vi "Periodic Tasks.vi"(8 "error in":errorcluster) -> ()   [LabVIEW 2020]
doc: "This VI runs in parallel to other tasks. It can contain as many user-defined periodic loops as you need. These can carry out PID or other sorts of timed response."
uses:
  <vilib>/Rock Robotics/WPI/Utilities/WPI_GetSetVariantRefNum.vi
  Robot sans CAN/MyGlobal.vi
  <vilib>/Rock Robotics/Network Tables/NT Write Numeric Array.vi
panel:
  out "force moteurs lance balle":dbl
  out "force feed balle":dbl
  out "ramasse balle":dbl
  out "Deploiement ramasse balle":dbl
  out "winch":dbl
  out "winch 2":dbl
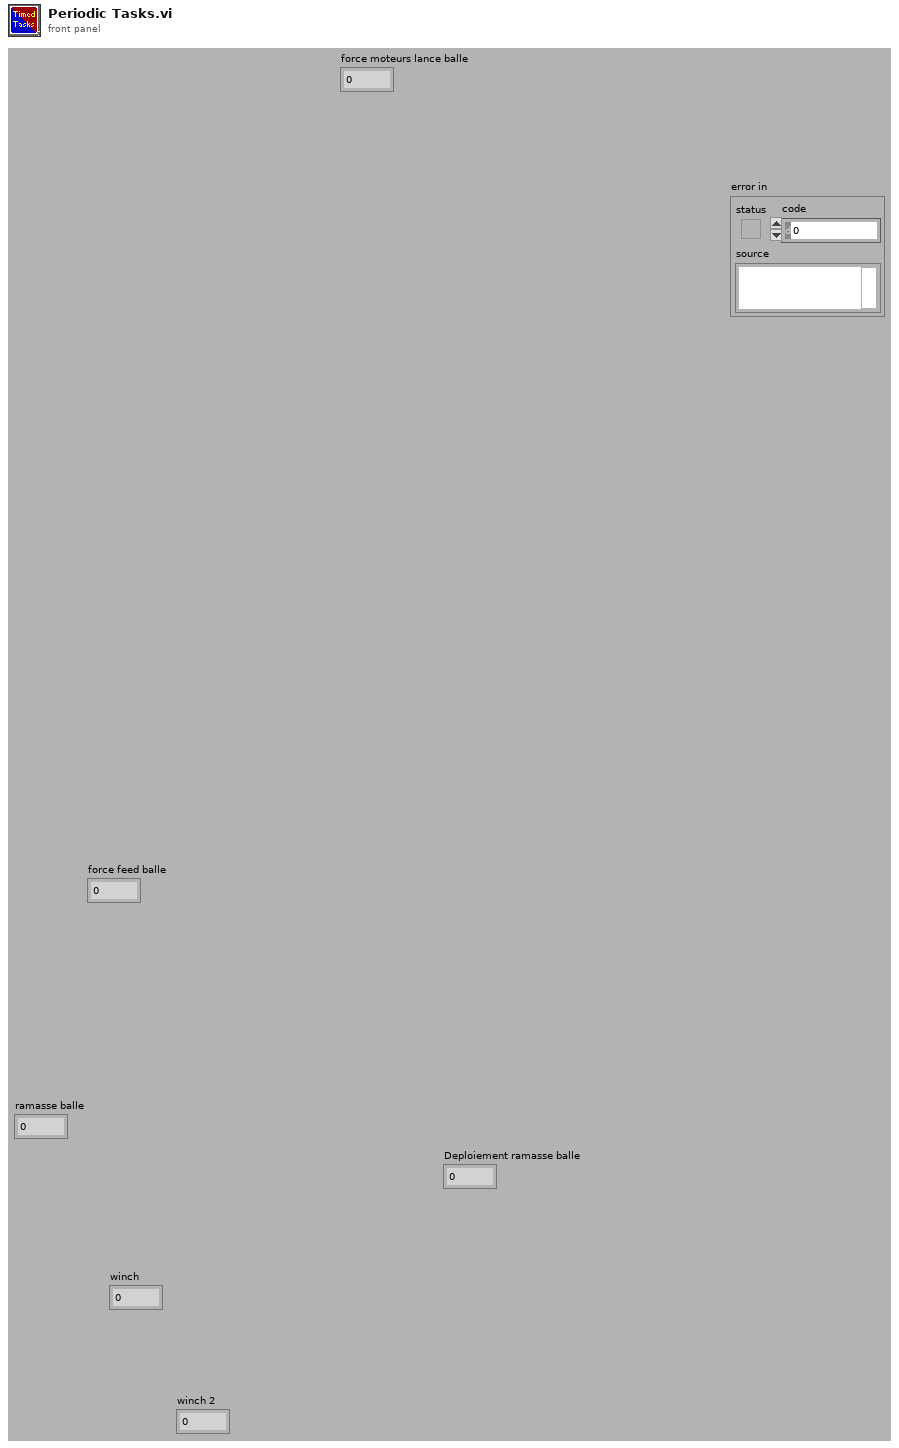
[diagram p1: front panel]
types:
  T1 = typedef "WPI_JoystickDevRef.ctl" = cluster{"Device":T2}
  T2 = typedef "WPI_JoystickDeviceEnum.ctl" = enum16{"USB 0", "USB 1", "USB 2", "USB 3", "USB 4", "USB 5"}
  T3 = typedef "WPI_RobotDriveDevRef.ctl" = cluster{"DevStatus":errorcluster, "Motors[]":T4[], "Square Inputs":bool, "Max Output":dbl}
  T4 = typedef "WPI_MotorControlDeviceRef.ctl" = cluster{"DeviceStatus":errorcluster, "Type":T5, "PWM":cluster{"PWM Channel":T6, "DeadBand":T7}, "CAN":cluster{"Device Number":u8, "SetOutput VI Ref":variant, "GetOutput VI Ref":variant, "Enable VI Ref":variant, "Disable VI Ref":variant, "Data":variant}, "Invert":bool, "DIO PWM":cluster{"PWM \"Enable\" Channel":T6, "DIOChannel":T8, "PWM Rate":dbl}}
  T5 = typedef "WPI_MotorControlType.ctl" = enum16{"PWM", "CAN", "DIO PWM"}
  T6 = typedef "FPGA_DIOPWMChannel.ctl" = enum8{"PWM 0", "PWM 1", "PWM 2", "PWM 3", "PWM 4", "PWM 5", "PWM 6", "PWM 7", "PWM 8", "PWM 9", "PWM MXP 0", "PWM MXP 1", "PWM MXP 2", "PWM MXP 3", "PWM MXP 4", "PWM MXP 5", "PWM MXP 6", "PWM MXP 7", "PWM MXP 8", "PWM MXP 9", "Invalid"}
  T7 = typedef "WPI_PWMDeadband.ctl" = cluster{"Name":string, "maxPositivePwm":i32, "minPositivePwm":i32, "centerPwm":i32, "maxNegativePwm":i32, "minNegativePwm":i32, "angularRange":u16}
  T8 = typedef "FPGA_DIOChannel.ctl" = enum8{"DIO 0", "DIO 1", "DIO 2", "DIO 3", "DIO 4", "DIO 5", "DIO 6", "DIO 7", "DIO 8", "DIO 9", "DIO MXP 0", "DIO MXP 1", "DIO MXP 2", "DIO MXP 3", "DIO MXP 4", "DIO MXP 5", "DIO MXP 6", "DIO MXP 7", "DIO MXP 8", "DIO MXP 9", "DIO MXP 10", "DIO MXP 11", "DIO MXP 12", "DIO MXP 13", "DIO MXP 14", "DIO MXP 15", "SPI Port CS1", "SPI Port CS2", "SPI Port CS3", "SPI Port MISO", "SPI Port MOSI", "Invalid"}
  T9 = cluster{"JoystickDevRef":T1, "RobotDriveDevRef":T3}
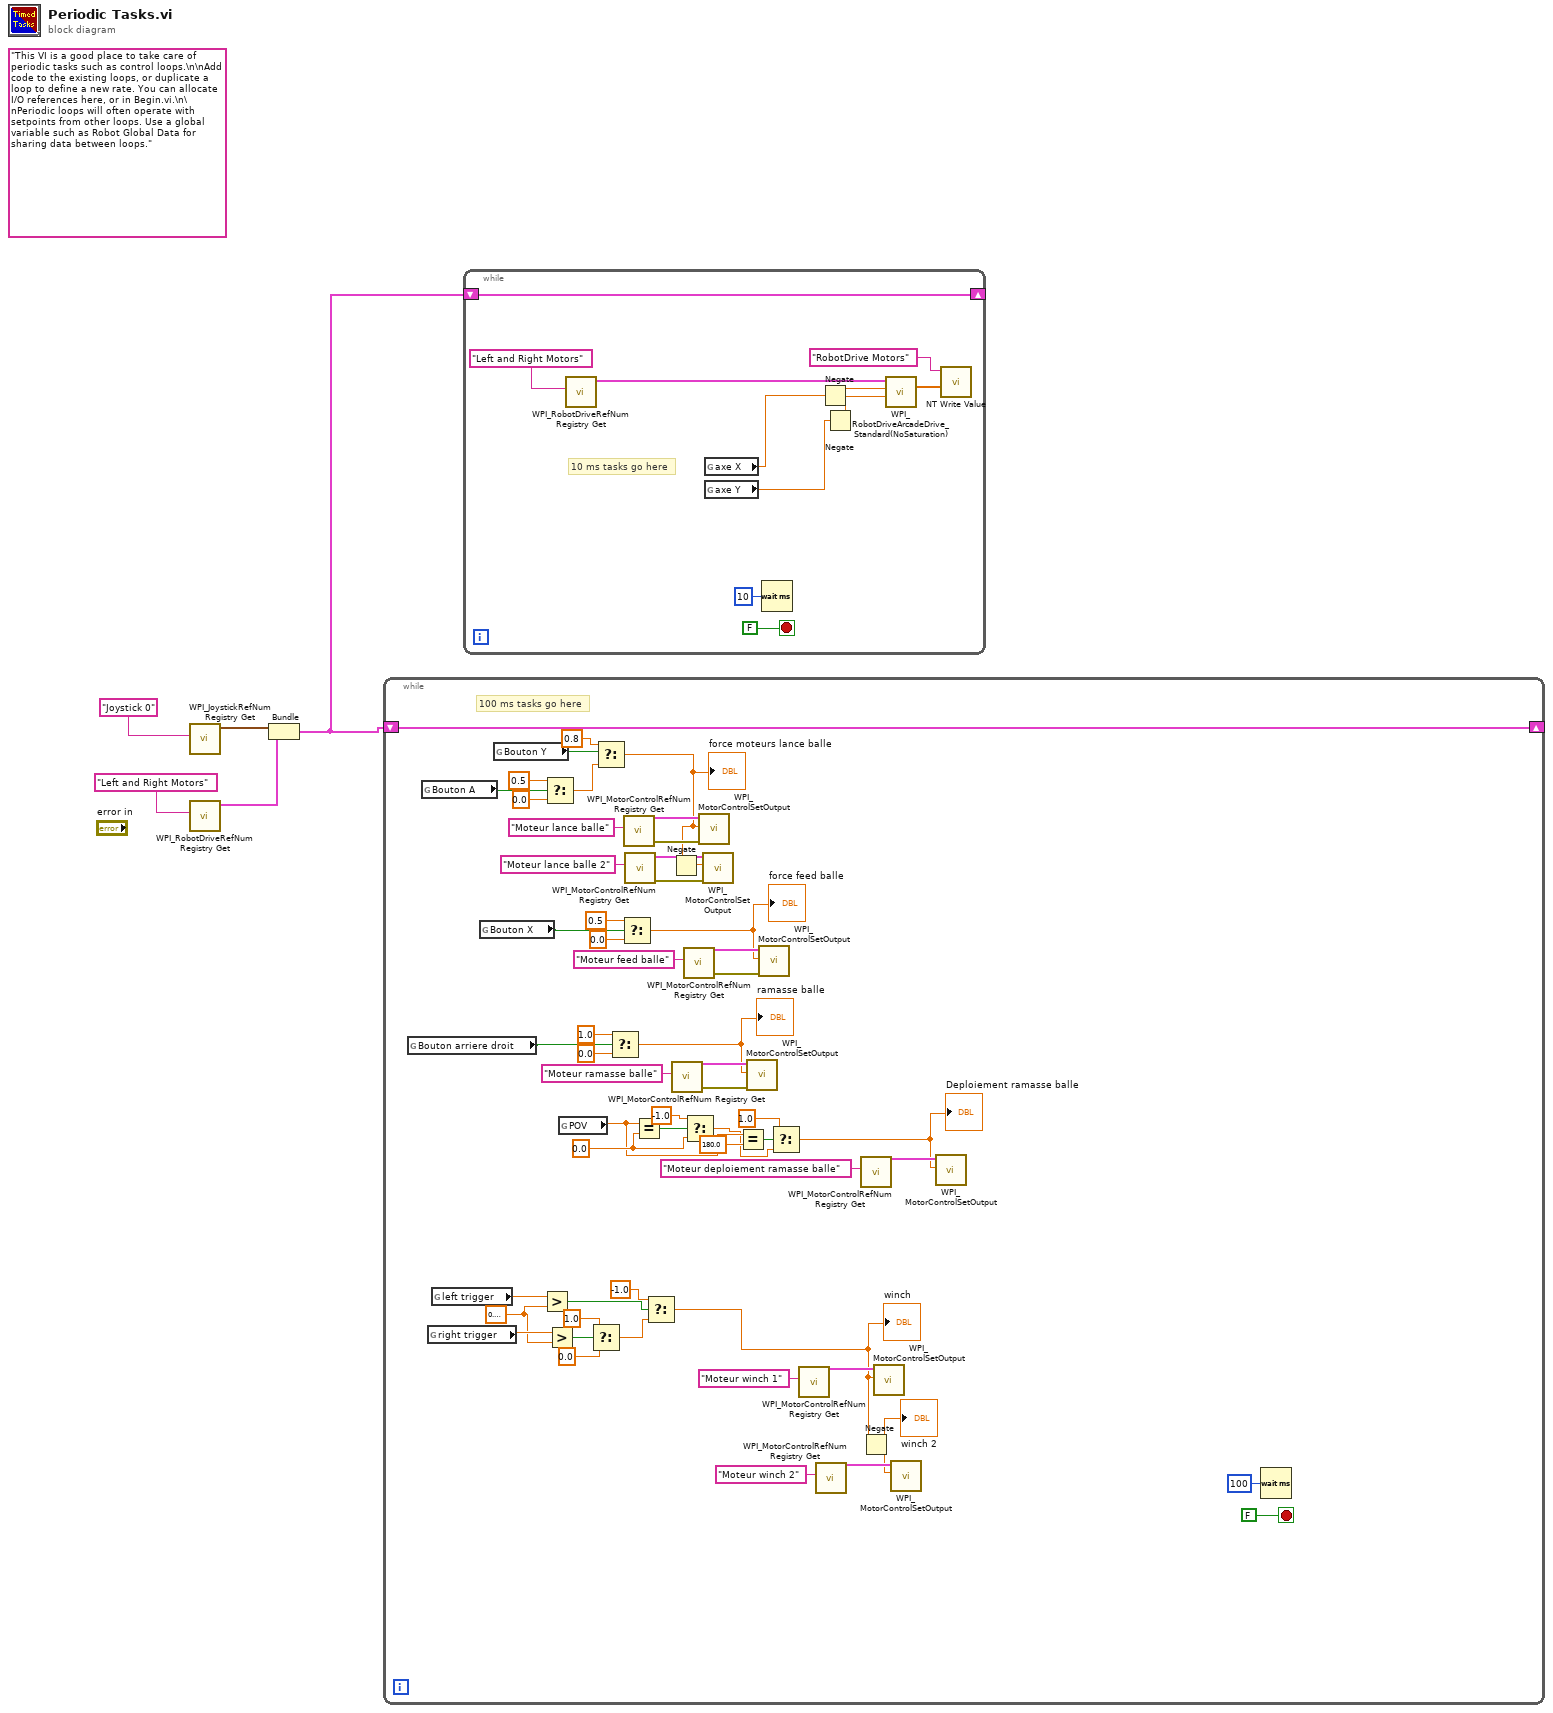
[diagram p0: block diagram]
diagram:
  (unwired) "This VI is a good place to take care of periodic tasks such as control loops.\n\nAdd code to the existing loops, or duplicate a loop to define a new rate. You can allocate I/O references here, or in Begin.vi.\n\nPeriodic loops will often operate with setpoints from other loops. Use a global variable such as Robot Global Data for sharing data between loops."
  n1 = call <vilib>:"WPI_JoystickRefNum Registry Get.vi"("refnum name"="Joystick 0") -> ("JoystickDevRef"=w3:T1)  [unwired: 1 in, 9 out]
  n2 = call <vilib>:"WPI_RobotDriveRefNum Registry Get.vi"("refnum name"="Left and Right Motors") -> ("RobotDriveDevRef"=w2:T3)  [unwired: 1 in, 9 out]
  n3 = Bundle("JoystickDevRef"=w3, "RobotDriveDevRef"=w2) -> (w1:T9)  [unwired: 1 out]
  n4 = while {
    shift-right: [w60] -> _
    shift-left: w1 -> [w60]
    stop <- FALSE stop-if-true
    w18 = sgl 0.2 ("y")
    w29 = 0.0
    # "100 ms tasks go here"
    n5 = global read "MyGlobal.vi" "Bouton arriere droit"() -> (w32:bool)
    n6 = global read "MyGlobal.vi" "Bouton A"() -> (w59:bool)
    n7 = global read "MyGlobal.vi" "right trigger"() -> (w19:sgl)
    n8 = global read "MyGlobal.vi" "left trigger"() -> (w20:sgl)
    n9 = global read "MyGlobal.vi" "Bouton X"() -> (w43:bool)
    n10 = global read "MyGlobal.vi" "Bouton Y"() -> (w55:bool)
    n11 = Greater?(x=w20, y=w18) -> (0:w15:bool)
    n12 = Select(t=0.5, s=w59, f=0.0) -> (s? t:f=w54:dbl)
    n13 = Greater?(x=w19, y=w18) -> (0:w17:bool)
    n14 = global read "MyGlobal.vi" "POV"() -> (w27:sgl)
    n15 = Select(t=1.0, s=w17, f=0.0) -> (s? t:f=w16:dbl)
    n16 = Select(t=0.8, s=w55, f=w54) -> (s? t:f=w47:dbl)
    "force moteurs lance balle" <- w47
    n17 = Select(t=1.0, s=w32, f=0.0) -> (s? t:f=w33:dbl)
    "ramasse balle" <- w33
    n18 = Select(t=0.5, s=w43, f=0.0) -> (s? t:f=w39:dbl)
    "force feed balle" <- w39
    n19 = call <vilib>:"WPI_MotorControlRefNum Registry Get.vi"("refnum name"="Moteur lance balle") -> ("error out"=w50:errorcluster, "MotorControlDevRef"=w51:T4)  [unwired: 9 in]
    n20 = call <vilib>:"WPI_MotorControlRefNum Registry Get.vi"("refnum name"="Moteur lance balle 2") -> ("error out"=w48:errorcluster, "MotorControlDevRef"=w49:T4)  [unwired: 9 in]
    n21 = Equal?(x=w27, y=w29) -> (x = y?=w31:bool)
    n22 = Select(t=-1.0, s=w15, f=w16) -> (s? t:f=w7:dbl)
    "winch" <- w7
    n23 = Negate(x=w47) -> (-x=w46:dbl)
    n24 = call <vilib>:"WPI_MotorControlRefNum Registry Get.vi"("refnum name"="Moteur ramasse balle") -> ("error out"=w34:errorcluster, "MotorControlDevRef"=w35:T4)  [unwired: 9 in]
    n25 = call <vilib>:"WPI_MotorControlRefNum Registry Get.vi"("refnum name"="Moteur feed balle") -> ("error out"=w40:errorcluster, "MotorControlDevRef"=w41:T4)  [unwired: 9 in]
    n26 = Select(t=-1.0, s=w31, f=w29) -> (s? t:f=w24:dbl)
    n27 = call <vilib>:"WPI_MotorControlSetOutput.vi"("error in (no error)"=w50, "Output"=w47, "MotorControlDevRef"=w51) -> ()  [unwired: 6 in, 3 out]
    n28 = call <vilib>:"WPI_MotorControlSetOutput.vi"("error in (no error)"=w48, "Output"=w46, "MotorControlDevRef"=w49) -> ()  [unwired: 6 in, 3 out]
    n29 = Equal?(x=w27, y=sgl 180.0) -> (x = y?=w28:bool)
    n30 = call <vilib>:"WPI_MotorControlSetOutput.vi"("error in (no error)"=w34, "Output"=w33, "MotorControlDevRef"=w35) -> ()  [unwired: 6 in, 3 out]
    n31 = call <vilib>:"WPI_MotorControlSetOutput.vi"("error in (no error)"=w40, "Output"=w39, "MotorControlDevRef"=w41) -> ()  [unwired: 6 in, 3 out]
    n32 = Select(t=1.0, s=w28, f=w24) -> (s? t:f=w21:dbl)
    "Deploiement ramasse balle" <- w21
    n33 = call <vilib>:"WPI_MotorControlRefNum Registry Get.vi"("refnum name"="Moteur winch 1") -> ("MotorControlDevRef"=w10:T4)  [unwired: 9 in, 1 out]
    n34 = call <vilib>:"WPI_MotorControlRefNum Registry Get.vi"("refnum name"="Moteur winch 2") -> ("MotorControlDevRef"=w8:T4)  [unwired: 9 in, 1 out]
    n35 = call <vilib>:"WPI_MotorControlRefNum Registry Get.vi"("refnum name"="Moteur deploiement ramasse balle") -> ("MotorControlDevRef"=w22:T4)  [unwired: 9 in, 1 out]
    n36 = Negate(x=w7) -> (-x=w6:dbl)
    "winch 2" <- w6
    n37 = call <vilib>:"WPI_MotorControlSetOutput.vi"("Output"=w7, "MotorControlDevRef"=w10) -> ()  [unwired: 7 in, 3 out]
    n38 = call <vilib>:"WPI_MotorControlSetOutput.vi"("Output"=w6, "MotorControlDevRef"=w8) -> ()  [unwired: 7 in, 3 out]
    n39 = call <vilib>:"WPI_MotorControlSetOutput.vi"("Output"=w21, "MotorControlDevRef"=w22) -> ()  [unwired: 7 in, 3 out]
    n40 = Wait (ms)(milliseconds to wait=u32 100) -> ()  [unwired: 1 out]
  }
  n41 = while {
    shift-right: [w71] -> _
    shift-left: w1 -> [w71]
    stop <- FALSE stop-if-true
    # "10 ms tasks go here"
    n42 = call <vilib>:"WPI_RobotDriveRefNum Registry Get.vi"("refnum name"="Left and Right Motors") -> ("RobotDriveDevRef"=w69:T3)  [unwired: 1 in, 9 out]
    n43 = global read "MyGlobal.vi" "axe X"() -> (w64:sgl)
    n44 = global read "MyGlobal.vi" "axe Y"() -> (w63:sgl)
    n45 = Wait (ms)(milliseconds to wait=u32 10) -> ()  [unwired: 1 out]
    n46 = Negate(x=w64) -> (-x=w65:sgl)
    n47 = Negate(x=w63) -> (-x=w66:sgl)
    n48 = call <vilib>:"WPI_RobotDriveArcadeDrive_Standard(NoSaturation).vi"("Y axis value"=w66, "X axis value"=w65, "RobotDriveDevRef"=w69) -> ("Motor Values"=w68:dbl[])  [unwired: 1 in, 7 out]
    n49 = call-poly <vilib>:"NT Write Value.vi"("Numeric Array"=w68, "Name"="RobotDrive Motors") -> ()  [unwired: 9 in, 1 out]
  }
